vi "PDC_GetLiveImageData.vi"(6 "Resolution":cluster{"Width":u32, "Height":u32}, 7 "ColorType":enum16{"MONO", "COLOR"}(ring), 8 "error in (no error)":errorcluster, 9 "BitDepth":u32, 10 "ChildNo":u32, 11 "DeviceNo":u32) -> (0 "error out":errorcluster, 2 "ErrorCode":u32, 3 "ReturnValue":u32, 4 "Data(8Bit)":u8[](array[numeric]), 5 "Data(16Bit)":u16[](array[numeric]))   [LabVIEW 2015]
doc: "This VI retrieves the live image of the specified child device."
uses:
  PDCLIB.dll
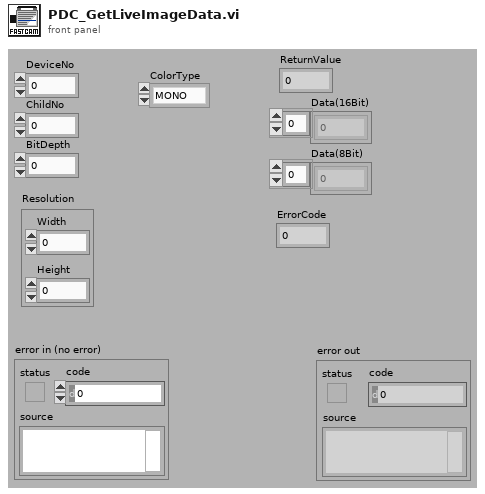
[diagram p1: front panel]
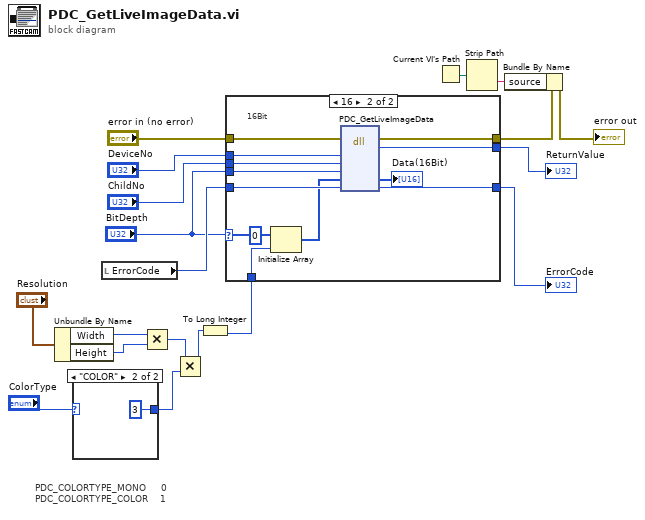
[diagram p0: block diagram]
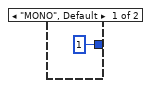
[diagram p2: hidden frame]
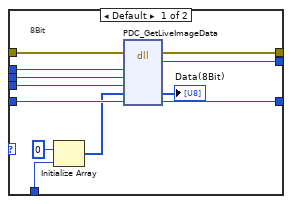
[diagram p3: hidden frame]
diagram:
  # "PDC_COLORTYPE_MONO\t\t\t\t\t0\nPDC_COLORTYPE_COLOR\t\t\t\t1"
  n1 = Unbundle By Name("Resolution") -> ("Width"=w8:u32, "Height"=w7:u32)
  n2 = case shown="\"COLOR\"" "ColorType" {
    tunnel: [u32 1 ("y") u32 3 ("y")] -> w11
    frame "MONO", Default {
    }
    frame "COLOR" {
    }
  }
  n3 = local read "ErrorCode"() -> (w17:u32)
  n4 = Multiply(x=w8, y=w7) -> (x*y=w12:u32)
  n5 = Multiply(x=w12, y=w11) -> (x*y=w10:u32)
  n6 = To Long Integer(number=w10) -> (32bit integer=w1:i32)
  n7 = case shown="16" "BitDepth" {
    tunnel: [w33 w45] -> w19
    tunnel: [w32 w44] -> w3
    tunnel: "error in (no error)" -> [w31 w43]
    tunnel: w17 -> [w30 w42]
    tunnel: "DeviceNo" -> [w29 w41]
    tunnel: "ChildNo" -> [w28 w40]
    tunnel: [w27 w39] -> w14
    tunnel: "BitDepth" -> [w26 w38]
    tunnel: w1 -> [w23 w35]
    frame Default {
      # "8Bit"
      n8 = Initialize Array(u8 0 ("—v‘f"), w23) -> (w22:u8[])
      n9 = dll-call lib="PDCLIB.dll" fn="PDC_GetLiveImageData"(error in=w31, "nDeviceNo"=w29, "nChildNo"=w28, "nBitDepth"=w26, "pData"=w22, "pErrorCode"=w30) -> (error out=w32:errorcluster, "return type"=w33:u32, "pData"=→"Data(8Bit)":u8[], "pErrorCode"=w27:u32)  [unwired: 5 in, 1 out]
    }
    frame 16 {
      # "16Bit"
      n10 = Initialize Array(u16 0 ("—v‘f"), w35) -> (w34:u16[])
      n11 = dll-call lib="PDCLIB.dll" fn="PDC_GetLiveImageData"(error in=w43, "nDeviceNo"=w41, "nChildNo"=w40, "nBitDepth"=w38, "pData"=w34, "pErrorCode"=w42) -> (error out=w44:errorcluster, "return type"=w45:u32, "pData"=→"Data(16Bit)":u16[], "pErrorCode"=w39:u32)  [unwired: 5 in, 1 out]
    }
  }
  "ReturnValue" <- w19
  "ErrorCode" <- w14
  n12 = Current VI's Path() -> (path=w4:path)
  n13 = Strip Path(path=w4) -> (name=w5:string)  [unwired: 1 out]
  n14 = Bundle By Name(cluster=w3, "source"=w5) -> (→"error out":errorcluster)
